vi "WS1021_MEMS Only 24DUT_Save Data_Ver1.0.vi"(0 "Header":string[](array[string]), 4 "File Name":string, 5 "error in (no error)":errorcluster, 6 "base path":path=path "C:/temp", 8 "Data In":string[](array[string])) -> (12 "Final":string[](array[string]), 19 "error out":errorcluster)   [LabVIEW 2017]
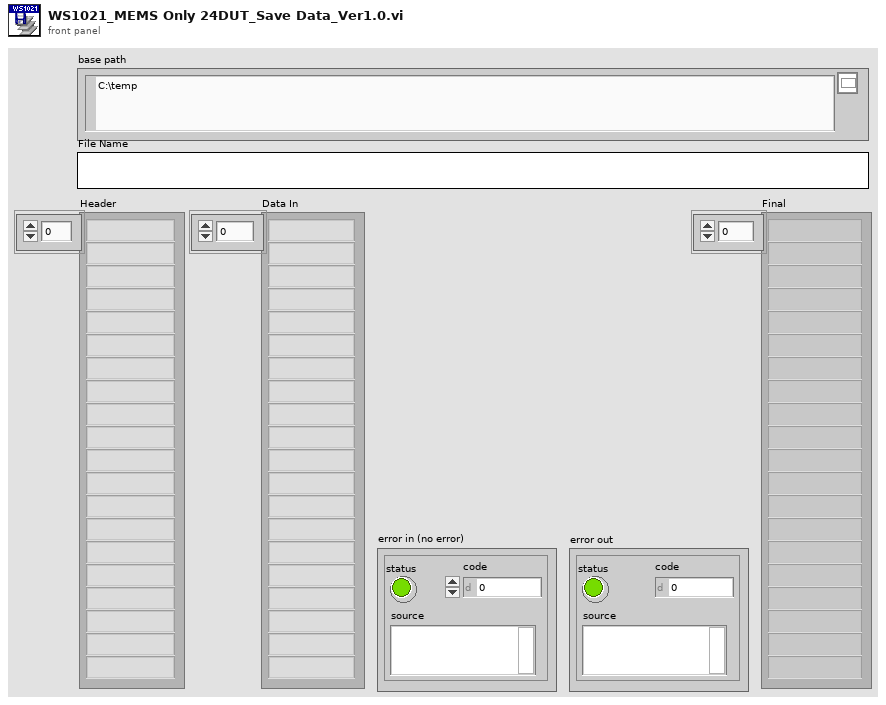
[diagram p1: front panel]
types:
  T1 = enum16{"open", "replace", "create", "open or create", "replace or create", "replace or create with confirmation"}
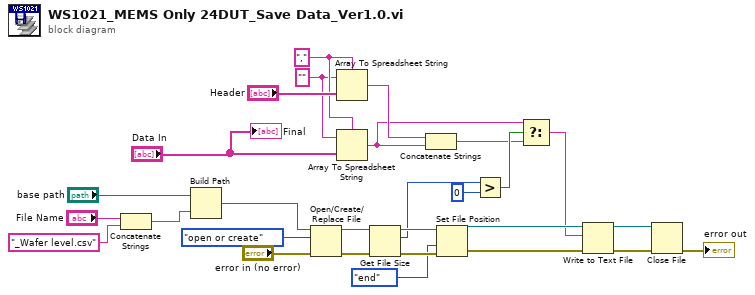
[diagram p0: block diagram]
diagram:
  w10 = "," ("delimiter (Tab)")
  w9 = "" ("format string")
  n1 = Concatenate Strings("File Name", "_Wafer level.csv" ("name or relative path")) -> (w3:string)
  n2 = Build Path(base path="base path", name or relative path=w3) -> (appended path=w27:path)
  n3 = Open/Create/Replace File(file path (use dialog)=w27, error in="error in (no error)", operation (0:open)=T1."open or create") -> (refnum out=w24:refnum<file>, error out=w25:errorcluster)  [unwired: 3 in, 1 out]
  n4 = Array To Spreadsheet String(delimiter (Tab)=w10, array="Header", 3:w9) -> (spreadsheet string=w14:string)
  n5 = Array To Spreadsheet String(delimiter (Tab)=w10, array="Data In", 3:w9) -> (spreadsheet string=w12:string)
  n6 = Get File Size(file=w24, error in=w25) -> (refnum out=w21:refnum<file>, size (in bytes)=w18:i64, 0:w23:errorcluster)
  n7 = Concatenate Strings(w14, w12) -> (w13:string)
  n8 = Set File Position(refnum=w21, from (0:start)=enum16{"start", "end", "current"}."end", error in=w23) -> (refnum out=w19:refnum<file>, error out=w20:errorcluster)  [unwired: 1 in]
  n9 = Greater?(x=w18, y=i64 0) -> (0:w16:bool)
  n10 = Select(t=w12, s=w16, f=w13) -> (s? t:f=w15:string)
  n11 = Write to Text File(file (use dialog)=w19, text=w15, error in=w20) -> (refnum out=w6:refnum<file>, error out=w7:errorcluster)  [unwired: 1 in, 1 out]
  n12 = Close File(refnum=w6, error in=w7) -> (error out=→"error out":errorcluster)  [unwired: 1 out]
  "Final" <- "Data In"
